vi "RUN-STOP-SING SEQ.vi"(0 "VISA":refnum<visa-resource-name>="GPIB0::1::INSTR", 1 "ACQUIRE":enum32{"RUN", "SINGLE SEQ"}(radio)) -> ()   [LabVIEW 2011]
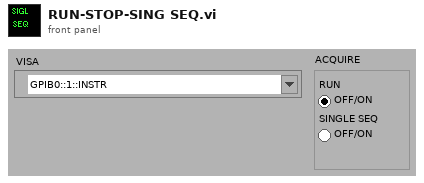
[diagram p1: front panel]
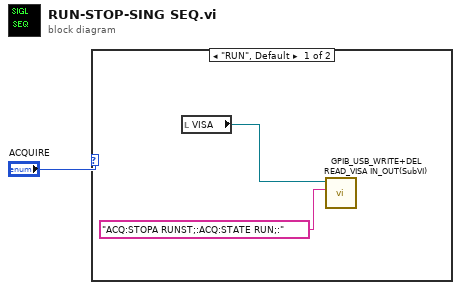
[diagram p0: block diagram]
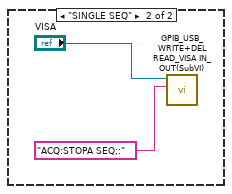
[diagram p2: hidden frame]
diagram:
  n1 = case shown="\"RUN\", Default" "ACQUIRE" {
    frame "RUN", Default {
      n2 = local read "VISA"() -> (w3:refnum<visa-resource-name>)
      n3 = call "GPIB_USB_WRITE+DEL READ_VISA IN_OUT(SubVI).vi"("VISA resource IN"=w3, "GPIB/USB WRITE"="ACQ:STOPA RUNST;:ACQ:STATE RUN;:") -> ()  [unwired: 4 in, 3 out]
    }
    frame "SINGLE SEQ" {
      n4 = call "GPIB_USB_WRITE+DEL READ_VISA IN_OUT(SubVI).vi"("VISA resource IN"="VISA", "GPIB/USB WRITE"="ACQ:STOPA SEQ;:") -> ()  [unwired: 4 in, 3 out]
    }
  }
